vi "Open Data Stream Call By VIs.vi"(11 "App Path":path) -> (2 "AI RT FIFO Ref":refnum<vi>, 3 "TCP Stream PC Ref":refnum<vi>)   [LabVIEW 2019]
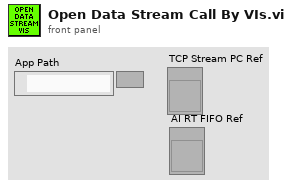
[diagram p1: front panel]
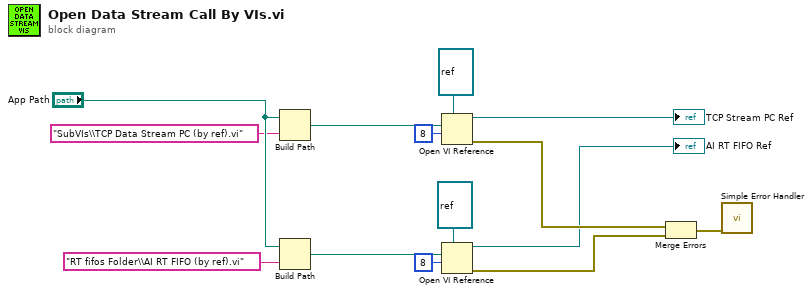
[diagram p0: block diagram]
diagram:
  n1 = Build Path(base path="App Path", name or relative path="SubVIs\\TCP Data Stream PC (by ref).vi") -> (appended path=w13:path)
  n2 = Build Path(base path="App Path", name or relative path="RT fifos Folder\\AI RT FIFO (by ref).vi") -> (appended path=w11:path)
  n3 = Open VI Reference(type specifier VI Refnum (for type only)=refnum<vi> refnum ("reference"), vi path=w13, options=8) -> (vi reference=→"TCP Stream PC Ref":refnum<vi>, error out=w8:errorcluster)  [unwired: 3 in]
  n4 = Open VI Reference(type specifier VI Refnum (for type only)=refnum<vi> refnum ("AI RT FIFO Ref"), vi path=w11, options=8) -> (vi reference=→"AI RT FIFO Ref":refnum<vi>, error out=w2:errorcluster)  [unwired: 3 in]
  n5 = Merge Errors(w8, w2) -> (w1:errorcluster)
  n6 = call <vilib>:"Simple Error Handler.vi"("error in (no error)"=w1) -> ()  [unwired: 4 in, 5 out]
